vi "Calculate Drift.vi"(2 "ADI IMU Interrupt DevRef":T1={"SimpleGyroDevRef"={"DevStatus"={"status"=FALSE, "code"=0, "source"=""}, "Handle"=0, "SPI Bus"=enum."SPI On-Board, CS0", "Device Found"=FALSE, "Sample Rate"=0.0, "Device Ready"=FALSE, "Yaw Axis"=enum."Z", "AHRS Algorithm"=enum."Complementary"}, "InterruptRef"={"DevStatus"={"status"=FALSE, "code"=0, "source"=""}, "InterruptIndex"=enum."0"}} {"SimpleGyroDevRef"."Sample Rate" min=0.25 max=100.0 step=0.25}) -> (0 "Drifts":T6, 1 "ADI IMU Interrupt DevRef Out":T1={"SimpleGyroDevRef"={"DevStatus"={"status"=FALSE, "code"=0, "source"=""}, "Handle"=0, "SPI Bus"=enum."SPI On-Board, CS0", "Device Found"=FALSE, "Sample Rate"=0.0, "Device Ready"=FALSE, "Yaw Axis"=enum."Z", "AHRS Algorithm"=enum."Complementary"}, "InterruptRef"={"DevStatus"={"status"=FALSE, "code"=0, "source"=""}, "InterruptIndex"=enum."0"}} {"SimpleGyroDevRef"."Sample Rate" min=0.25 max=100.0 step=0.25})   [LabVIEW 2015]
uses:
  ADI MXP IMU/WPI_AnalogDevicesIMUInterruptDevRef.ctl
  ADI MXP IMU/WPI_AnalogDevicesIMUDevRef.ctl
  <vilib>/Rock Robotics/SystemInterfaces/spilib/spi_bus.ctl
  <vilib>/Rock Robotics/WPI/Interrupt/WPI_InterruptRef.ctl
  <vilib>/Rock Robotics/SystemInterfaces/Interrupt/FPGA_InterruptIndex.ctl
  ADI MXP IMU/FRC ADI MXP IMU.lvlib
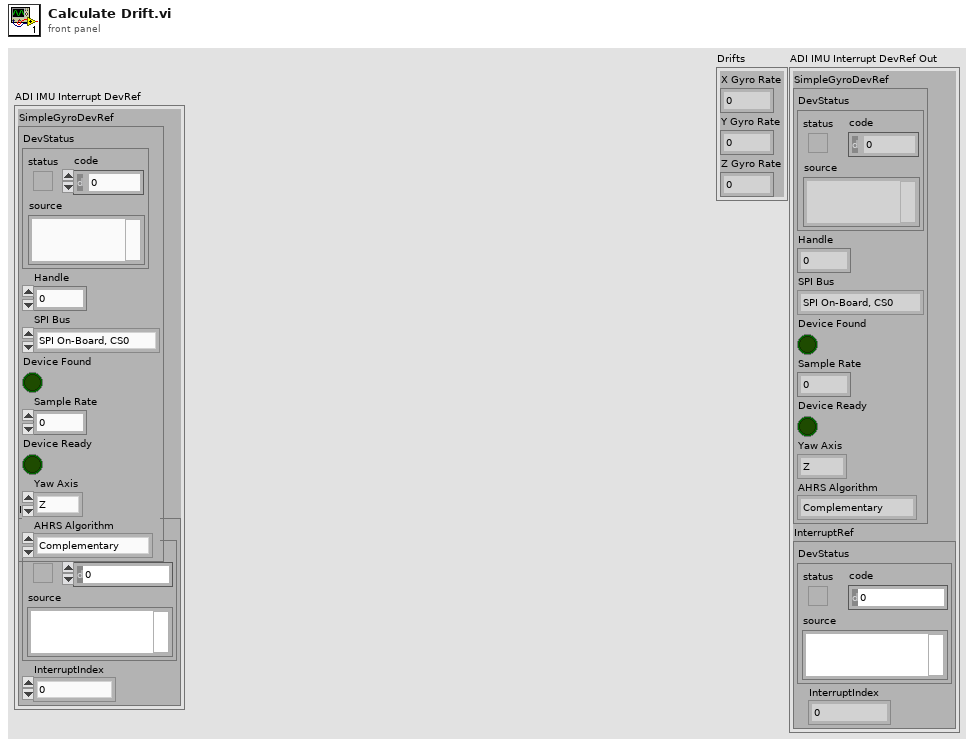
[diagram p1: front panel]
types:
  T1 = typedef "FRC ADI MXP IMU.lvlib/WPI_AnalogDevicesIMUInterruptDevRef.ctl" = cluster{"SimpleGyroDevRef":T2, "InterruptRef":T4}
  T2 = typedef "FRC ADI MXP IMU.lvlib/WPI_AnalogDevicesIMUDevRef.ctl" = cluster{"DevStatus":errorcluster, "Handle":i32, "SPI Bus":T3, "Device Found":bool, "Sample Rate":dbl, "Device Ready":bool, "Yaw Axis":enum16{"X", "Y", "Z"}, "AHRS Algorithm":enum16{"Complementary", "Madgwick"}}
  T3 = typedef "spi_bus.ctl" = enum16{"SPI On-Board, CS0", "SPI On-Board, CS1", "SPI On-Board, CS2", "SPI On-Board, CS3", "SPI MXP", "Invalid"}
  T4 = typedef "WPI_InterruptRef.ctl" = cluster{"DevStatus":errorcluster, "InterruptIndex":T5}
  T5 = typedef "FPGA_InterruptIndex.ctl" = enum8{"0", "1", "2", "3", "4", "5", "6", "7", "Invalid"}
  T6 = cluster{"X Gyro Rate":dbl, "Y Gyro Rate":dbl, "Z Gyro Rate":dbl}
  T7 = cluster{"X Gyro Rate":dbl, "Y Gyro Rate":dbl, "Z Gyro Rate":dbl, "X Accel":dbl, "Y Accel":dbl, "Z Accel":dbl, "X Mag":dbl, "Y Mag":dbl, "Z Mag":dbl, "Barometer":dbl, "Temperature":dbl}
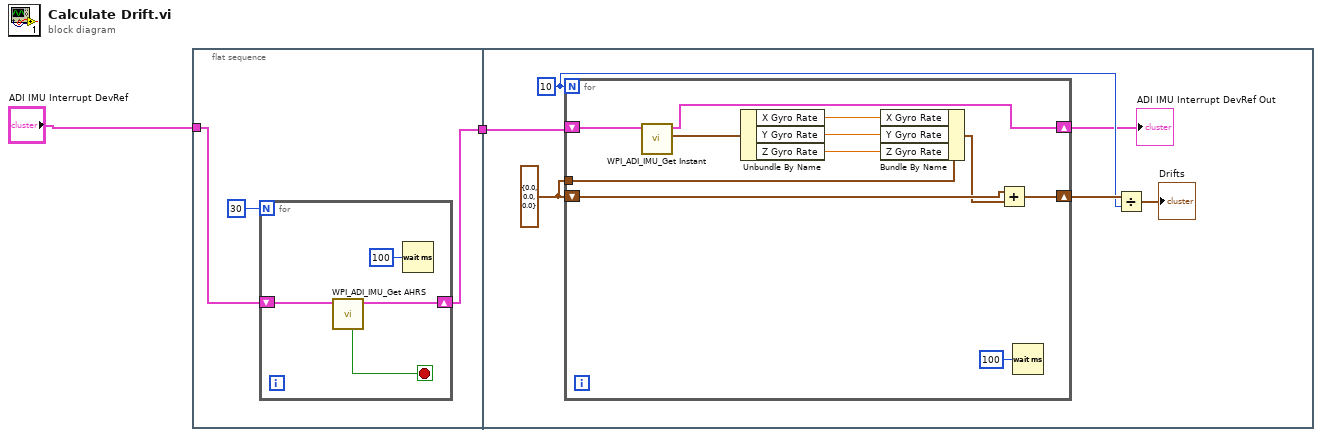
[diagram p0: block diagram]
diagram:
  n1 = flat-sequence {
    tunnel: "ADI IMU Interrupt DevRef" -> [w4]
    tunnel: [w3] -> w1
    tunnel: w1 -> [w11]
    frame #0 {
      n2 = for {
        N: 30 -> [_]
        shift-right: [w7] -> w3
        shift-left: w4 -> [w6]
        stop <- w9 stop-if-true
        n3 = call "WPI_ADI_IMU_Get AHRS.vi"("ADI IMU Interrupt DevRef"=w6) -> ("ADI IMU Interrupt DevRef Out"=w7:T1, "Sensor Ready Out"=w9:bool)  [unwired: 6 in, 3 out]
        n4 = Wait (ms)(milliseconds to wait=u32 100) -> ()  [unwired: 1 out]
      }
    }
    frame #1 {
      w15 = T6 {"X Gyro Rate"=0.0, "Y Gyro Rate"=0.0, "Z Gyro Rate"=0.0} ("input cluster")
      w13 = 10
      n5 = for {
        N: w13 -> [_]
        shift-right: [w17] -> w14
        shift-left: w15 -> [w19]
        tunnel: w15 -> [w21]
        shift-right: [w16] -> w10
        shift-left: w11 -> [w25]
        n6 = call "WPI_ADI_IMU_Get Instant.vi"("ADI IMU Interrupt DevRef"=w25) -> ("IMU Data"=w20:T7, "ADI IMU Interrupt DevRef Out"=w16:T1)  [unwired: 7 in, 2 out]
        n7 = Unbundle By Name(w20) -> ("X Gyro Rate"=w23:dbl, "Y Gyro Rate"=w24:dbl, "Z Gyro Rate"=w22:dbl)
        n8 = Bundle By Name(cluster=w21, "X Gyro Rate"=w23, "Y Gyro Rate"=w24, "Z Gyro Rate"=w22) -> (w18:T6)
        n9 = Add(x=w19, y=w18) -> (x+y=w17:T6)
        n10 = Wait (ms)(milliseconds to wait=u32 100) -> ()  [unwired: 1 out]
      }
      "ADI IMU Interrupt DevRef Out" <- w10
      n11 = Divide(x=w14, y=w13) -> (x/y=→"Drifts":T6)
    }
  }
